vi "RebuildCmdListing.vi"(3 "Params":cluster{"Constant":string, "value":string}[](array[cluster]), 4 "Contents":string, 5 "String in":string) -> (1 "array":string[](array[string]), 2 "String out":string)   [LabVIEW 2014]
panel:
  out "Contents 2":string
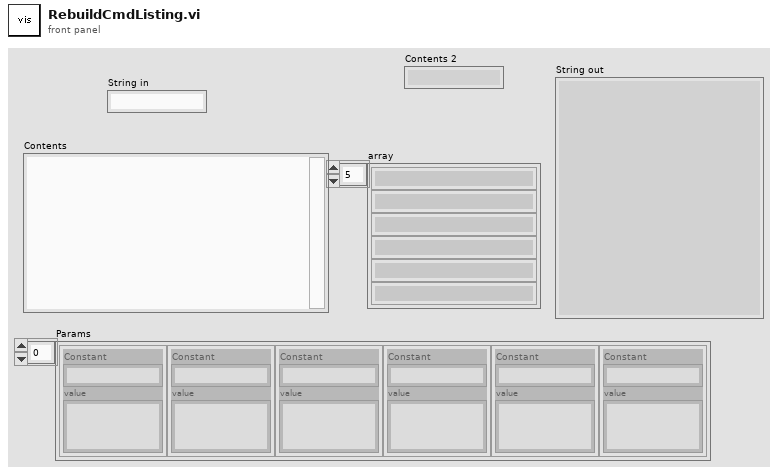
[diagram p1: front panel]
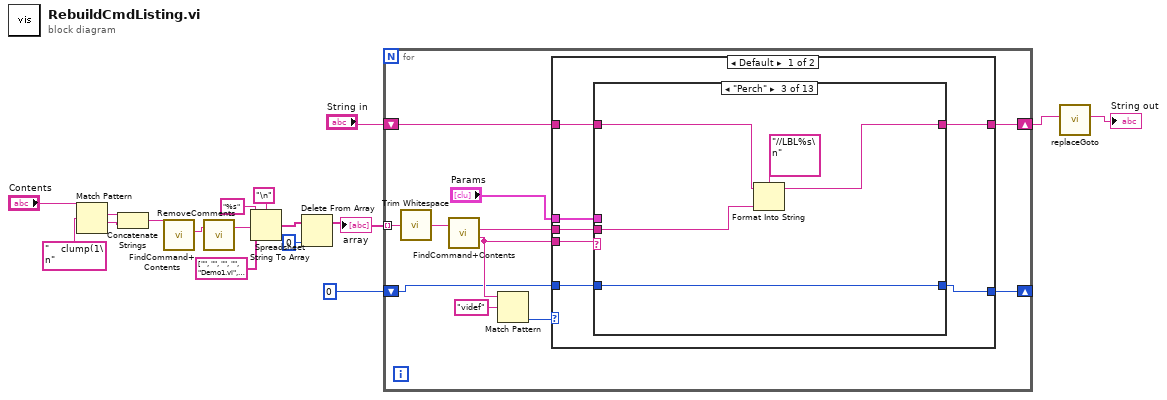
[diagram p0: block diagram]
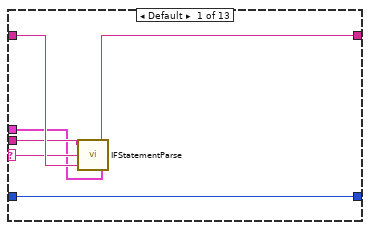
[diagram p2: hidden frame]
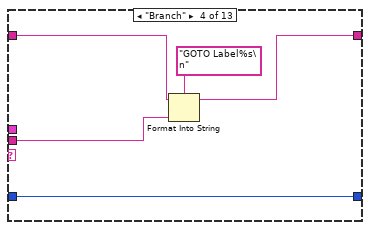
[diagram p4: hidden frame]
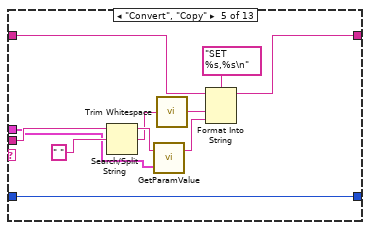
[diagram p5: hidden frame]
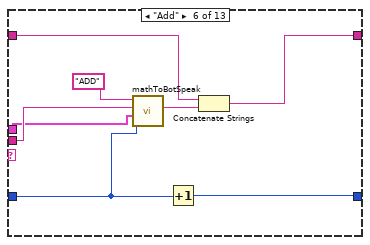
[diagram p6: hidden frame]
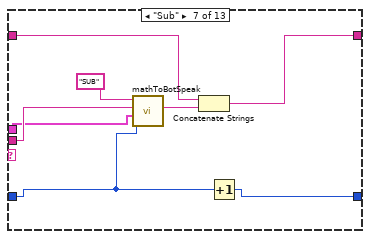
[diagram p7: hidden frame]
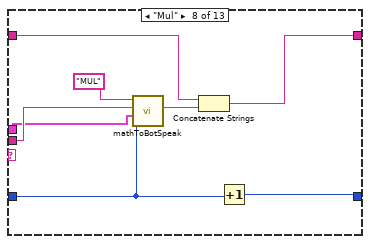
[diagram p8: hidden frame]
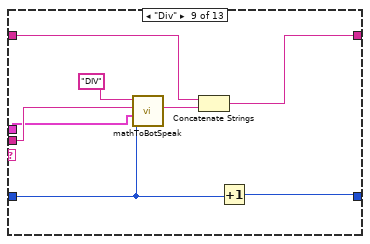
[diagram p9: hidden frame]
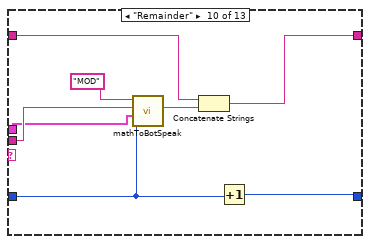
[diagram p10: hidden frame]
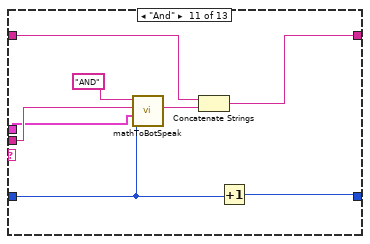
[diagram p11: hidden frame]
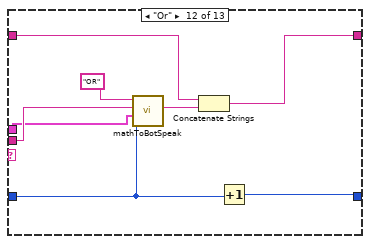
[diagram p12: hidden frame]
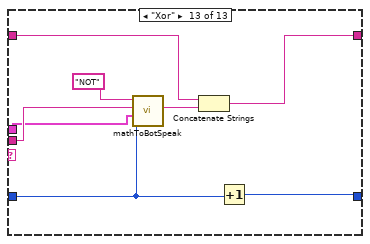
[diagram p13: hidden frame]
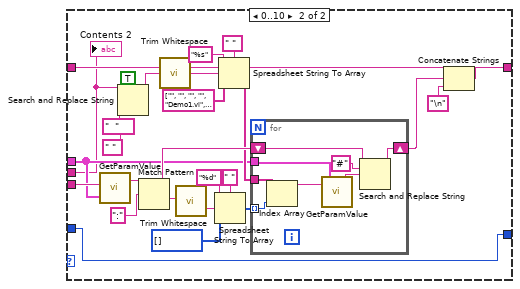
[diagram p14: hidden frame]
diagram:
  n1 = Match Pattern(string="Contents", regular expression="    clump(1\n") -> (match substring=w9:string, after substring=w10:string)  [unwired: 1 in, 2 out]
  n2 = Concatenate Strings(w9, w10) -> (w11:string)
  n3 = call <vilib>:"FindCommand+Contents.vi"("Via file in"=w11) -> ("Contents"=w12:string)  [unwired: 1 in, 3 out]
  n4 = call <vilib>:"RemoveComments.vi"("Via file in"=w12) -> ("Via file out"=w13:string)  [unwired: 2 in]
  n5 = Spreadsheet String To Array(delimiter (Tab)="\n", format string="%s", spreadsheet string=w13, array type (2D Dbl)=string[] ["", "", "", "", "Demo1.vi", "DigitalWrite.vi", "VS_Wait.vi", ""] ("Array 3")) -> (array=w16:string[])
  n6 = Delete From Array(array=w16, index=0) -> (array with subset deleted=w5:string[])  [unwired: 1 in, 1 out]
  "array" <- w5
  n7 = for {
    tunnel: w5 -> [w28] mode=indexing
    shift-right: [w25] -> w2
    shift-left: "String in" -> [w26]
    shift-right: [w18] -> _
    shift-left: 0 -> [w19]
    n8 = call <vilib>:"Trim Whitespace.vi"("string"=w28) -> ("trimmed string"=w27:string)  [unwired: 1 in]
    n9 = call <vilib>:"FindCommand+Contents.vi"("Via file in"=w27) -> ("Contents"=w23:string, "command"=w22:string)  [unwired: 1 in, 2 out]
    n10 = Match Pattern(string=w22, regular expression="videf") -> (offset past match=w20:i32)  [unwired: 1 in, 3 out]
    n11 = case shown="Default" w20 {
      tunnel: w22 -> [w35 w154]
      tunnel: w26 -> [w34 w141]
      tunnel: [w32 w140] -> w25
      tunnel: "Params" -> [w31 w137]
      tunnel: w23 -> [w33 w134]
      tunnel: w19 -> [w30 w129]
      tunnel: [w29 w129] -> w18
      frame Default {
        n12 = case shown="\"Perch\"" w35 {
          selector: w35 -> [w39 _ _ _ _ _ _ _ _ _ _ _ _]
          tunnel: w34 -> [w41 w43 w47 w52 w63 w68 w76 w84 w92 w100 w108 w116 w124]
          tunnel: w33 -> [w40 _ w46 w51 w61 w71 w79 w87 w95 w103 w111 w119 w127]
          tunnel: [w38 w43 w45 w50 w56 w67 w75 w83 w91 w99 w107 w115 w123] -> w32
          tunnel: w31 -> [w37 _ _ _ w60 w70 w78 w86 w94 w102 w110 w118 w126]
          tunnel: [w36 w42 w44 w49 w58 w66 w74 w82 w90 w98 w106 w114 w122] -> w29
          tunnel: w30 -> [w36 w42 w44 w49 w58 w65 w73 w81 w89 w97 w105 w113 w121]
          frame Default {
            n13 = call <vilib>:"IFStatementParse.vi"("Params"=w37, "BotSpeak in"=w41, "Command"=w39, "Contents"=w40) -> ("BotSpeak out"=w38:string)  [unwired: 1 in]
          }
          frame "" {
          }
          frame "Perch" {
            n14 = Format Into String(format string="//LBL%s\n", initial string=w47, w46) -> (resulting string=w45:string)  [unwired: 1 in, 1 out]
          }
          frame "Branch" {
            n15 = Format Into String(format string="GOTO Label%s\n", initial string=w52, w51) -> (resulting string=w50:string)  [unwired: 1 in, 1 out]
          }
          frame "Convert", "Copy" {
            n16 = Search/Split String(string=w61, search string/char (-)=" ") -> (substring before match=w59:string, match + rest of string=w55:string)  [unwired: 1 in, 1 out]
            n17 = call <vilib>:"GetParamValue.vi"("Params"=w60, "command"=w59) -> ("value"=w57:string)  [unwired: 1 in]
            n18 = call <vilib>:"Trim Whitespace.vi"("string"=w55) -> ("trimmed string"=w54:string)  [unwired: 1 in]
            n19 = Format Into String(format string="SET %s,%s\n", initial string=w63, w54, w57) -> (resulting string=w56:string)  [unwired: 1 in, 1 out]
          }
          frame "Add" {
            n20 = call <vilib>:"mathToBotSpeak.vi"("Numeric"=w65, "Params"=w70, "String in"=w71, "Command"="ADD") -> ("resulting string"=w69:string)  [unwired: 7 in]
            n21 = Increment(x=w65) -> (x+1=w66:i32)
            n22 = Concatenate Strings(w68, w69) -> (w67:string)
          }
          frame "Sub" {
            n23 = call <vilib>:"mathToBotSpeak.vi"("Numeric"=w73, "Params"=w78, "String in"=w79, "Command"="SUB") -> ("resulting string"=w77:string)  [unwired: 7 in]
            n24 = Concatenate Strings(w76, w77) -> (w75:string)
            n25 = Increment(x=w73) -> (x+1=w74:i32)
          }
          frame "Mul" {
            n26 = call <vilib>:"mathToBotSpeak.vi"("Numeric"=w81, "Params"=w86, "String in"=w87, "Command"="MUL") -> ("resulting string"=w85:string)  [unwired: 7 in]
            n27 = Concatenate Strings(w84, w85) -> (w83:string)
            n28 = Increment(x=w81) -> (x+1=w82:i32)
          }
          frame "Div" {
            n29 = call <vilib>:"mathToBotSpeak.vi"("Numeric"=w89, "Params"=w94, "String in"=w95, "Command"="DIV") -> ("resulting string"=w93:string)  [unwired: 7 in]
            n30 = Concatenate Strings(w92, w93) -> (w91:string)
            n31 = Increment(x=w89) -> (x+1=w90:i32)
          }
          frame "Remainder" {
            n32 = call <vilib>:"mathToBotSpeak.vi"("Numeric"=w97, "Params"=w102, "String in"=w103, "Command"="MOD") -> ("resulting string"=w101:string)  [unwired: 7 in]
            n33 = Concatenate Strings(w100, w101) -> (w99:string)
            n34 = Increment(x=w97) -> (x+1=w98:i32)
          }
          frame "And" {
            n35 = call <vilib>:"mathToBotSpeak.vi"("Numeric"=w105, "Params"=w110, "String in"=w111, "Command"="AND") -> ("resulting string"=w109:string)  [unwired: 7 in]
            n36 = Concatenate Strings(w108, w109) -> (w107:string)
            n37 = Increment(x=w105) -> (x+1=w106:i32)
          }
          frame "Or" {
            n38 = call <vilib>:"mathToBotSpeak.vi"("Numeric"=w113, "Params"=w118, "String in"=w119, "Command"="OR") -> ("resulting string"=w117:string)  [unwired: 7 in]
            n39 = Concatenate Strings(w116, w117) -> (w115:string)
            n40 = Increment(x=w113) -> (x+1=w114:i32)
          }
          frame "Xor" {
            n41 = call <vilib>:"mathToBotSpeak.vi"("Numeric"=w121, "Params"=w126, "String in"=w127, "Command"="NOT") -> ("resulting string"=w125:string)  [unwired: 7 in]
            n42 = Concatenate Strings(w124, w125) -> (w123:string)
            n43 = Increment(x=w121) -> (x+1=w122:i32)
          }
        }
      }
      frame 0..10 {
        n44 = call <vilib>:"GetParamValue.vi"("Params"=w137, "command"=w154) -> ("value"=w153:string)  [unwired: 1 in]
        n45 = Search and Replace String(replace all?=TRUE ("replace all? (F)"), input string=w134, search string="  ", replace string=" " ("replace string (\"\")")) -> (result string=w130:string)  [unwired: 4 in, 3 out]
        n46 = Match Pattern(string=w153, regular expression=":") -> (before substring=w144:string, after substring=w151:string)  [unwired: 1 in, 2 out]
        n47 = call <vilib>:"Trim Whitespace.vi"("string"=w130) -> ("trimmed string"=w135:string)  [unwired: 1 in]
        n48 = call <vilib>:"Trim Whitespace.vi"("string"=w151) -> ("trimmed string"=w136:string)  [unwired: 1 in]
        n49 = Spreadsheet String To Array(delimiter (Tab)=" ", format string="%d", spreadsheet string=w136, array type (2D Dbl)=i32[] [] ("Array 3")) -> (array=w142:i32[])
        n50 = Spreadsheet String To Array(delimiter (Tab)=" ", format string="%s", spreadsheet string=w135, array type (2D Dbl)=string[] ["", "", "", "", "Demo1.vi", "DigitalWrite.vi", "VS_Wait.vi", ""] ("Array 3")) -> (array=w143:string[])
        n51 = for {
          shift-right: [w161] -> w139
          shift-left: w144 -> [w162]
          tunnel: w143 -> [w159]
          tunnel: w142 -> [w158] mode=indexing
          tunnel: w137 -> [w157]
          n52 = Index Array(array=w159, index=w158) -> (element=w156:string)
          n53 = call <vilib>:"GetParamValue.vi"("Params"=w157, "command"=w156) -> ("value"=w155:string)  [unwired: 1 in]
          n54 = Search and Replace String(input string=w162, search string="#", replace string=w155) -> (result string=w161:string)  [unwired: 5 in, 3 out]
        }
        n55 = Concatenate Strings(w141, w139, "\n" ("delimiter (Tab)")) -> (w140:string)
        "Contents 2" <- w134
      }
    }
  }
  n56 = call <vilib>:"replaceGoto.vi"("String in"=w2) -> ("BotSpeak Out"=→"String out":string)  [unwired: 10 in]
